vi "Write DER SetPointP DVR.vi"(8 "error in":errorcluster, 10 "DER_SetPointP":T1, 11 "EMS Generic in":refnum<class "EMS Generic.lvclass">) -> (0 "error out":errorcluster, 3 "EMS Generic out":refnum<class "EMS Generic.lvclass">)   [LabVIEW 2018, in "EMS Generic Actor.lvlib" / "EMS Generic.lvclass"]
uses:
  EMS Generic.lvclass
  <vilib>/ORNL/CSEISMIC DDS/CSEISMIC DDS Base/Data Types/DER_SetPointP.ctl
  <vilib>/ORNL/CSEISMIC DDS/CSEISMIC DDS Base/Data Types/Controls/DeviceID.ctl
  EMS Generic.lvclass/EMS Generic.ctl
  <vilib>/ORNL/CSEISMIC DDS/CSEISMIC DDS Base/CSEISMIC DDS.lvclass
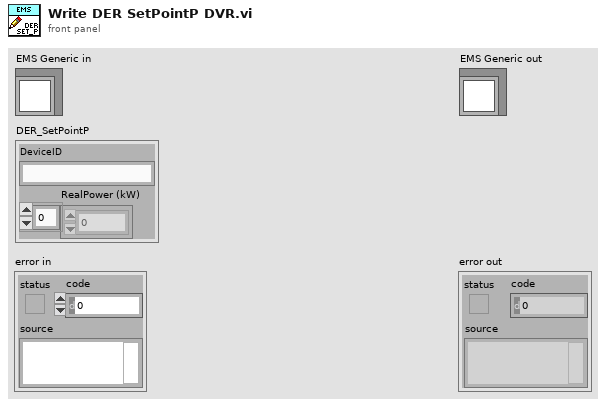
[diagram p1: front panel]
types:
  T1 = typedef "CSEISMIC DDS.lvlib/CSEISMIC DDS.lvclass/DER_SetPointP.ctl" = cluster{"DeviceID":T2, "RealPower (kW)":dbl[]}
  T2 = typedef "CSEISMIC DDS.lvlib/CSEISMIC DDS.lvclass/DeviceID.ctl" = string
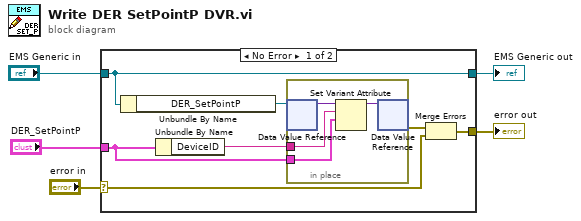
[diagram p0: block diagram]
diagram:
  n1 = case shown="No Error" "error in" {
    selector: "error in" -> [w12 w18]
    tunnel: [w7 w18] -> w4
    tunnel: [w11 w17] -> w2
    tunnel: "EMS Generic in" -> [w11 w17]
    tunnel: "DER_SetPointP" -> [w9 _]
    frame No Error {
      n2 = Unbundle By Name(w11) -> ("DER_SetPointP"=w8:refnum<data-value>)
      n3 = Unbundle By Name(w9) -> ("DeviceID"=w10:T2)
      n4 = in-place {
        in-place-border: w10 -> [w14]
        in-place-border: w9 -> [w13]
        n5 = in-place-dvr #1(w8) -> (w16:variant)  [unwired: 1 out]
        n6 = Set Variant Attribute(Variant=w16, name=w14, value=w13) -> (Variant out=w15:variant)  [unwired: 1 in, 2 out]
        n7 = in-place-dvr #1(w15) -> (w6:errorcluster)  [unwired: 1 out]
      }
      n8 = Merge Errors(w6, w12) -> (w7:errorcluster)
    }
    frame Error {
    }
  }
  "error out" <- w4
  "EMS Generic out" <- w2
